vi "Two Separare Slopes Using Sub VI.vi"() -> ()   [LabVIEW 2012]
panel:
  in  "Slope 2 Y2":dbl
  in  "Slope 2 X2":dbl
  in  "Slope 2 Y1":dbl
  in  "Slope 2 X1":dbl
  in  "Slope 1 Y2":dbl
  in  "Slope 1 X2":dbl
  in  "Slope 1 Y1":dbl
  in  "Slope 1 X1":dbl
  out "Slope 2":dbl
  out "Slope 1":dbl
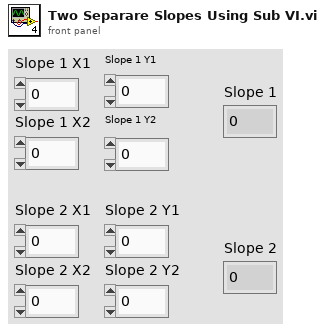
[diagram p1: front panel]
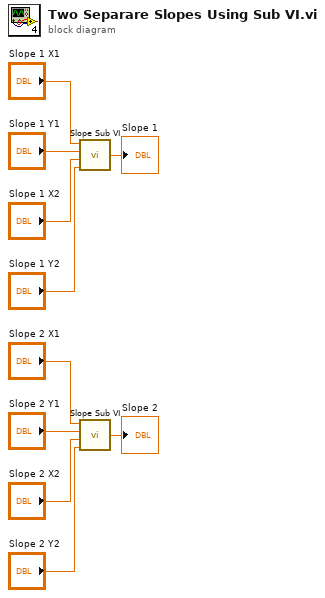
[diagram p0: block diagram]
diagram:
  n1 = call "Slope Sub VI.vi"("Y2"="Slope 1 Y2", "X2"="Slope 1 X2", "Y1"="Slope 1 Y1", "X1"="Slope 1 X1") -> ("Slope"=→"Slope 1":dbl)
  n2 = call "Slope Sub VI.vi"("Y2"="Slope 2 Y2", "X2"="Slope 2 X2", "Y1"="Slope 2 Y1", "X1"="Slope 2 X1") -> ("Slope"=→"Slope 2":dbl)
